vi "GOOP_DebugLogger.vi"(6 "ActivateDon'tCloseVI":bool, 7 "ActivateDebugging":bool, 8 "error in (no error)":errorcluster, 10 "Data":string, 11 "State":string) -> (0 "error out":errorcluster, 1 "Don'tCloseVI":bool, 3 "Debugging":bool)   [LabVIEW 2020]
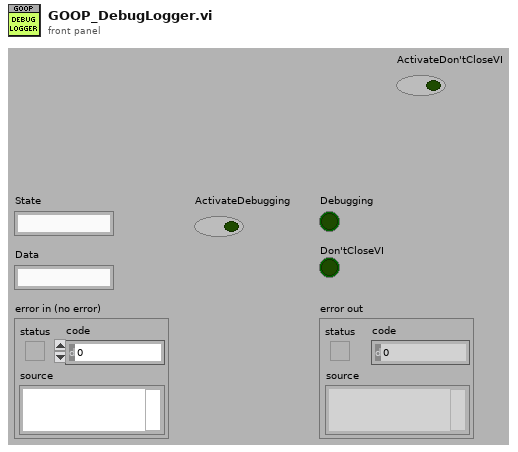
[diagram p1: front panel]
types:
  T1 = enum16{"open", "replace", "create", "open or create", "replace or create", "replace or create with confirmation"}
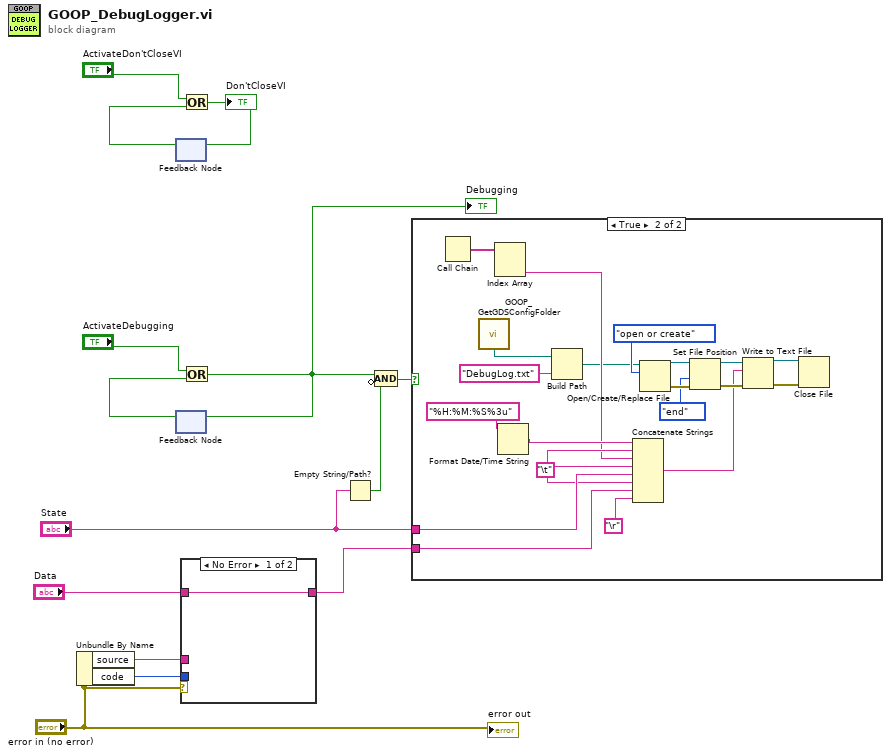
[diagram p0: block diagram]
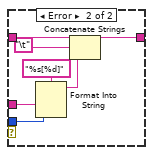
[diagram p2: hidden frame]
diagram:
  n1 = Unbundle By Name("error in (no error)") -> ("source"=w9:string, "code"=w8:i32)
  n2 = feedback #1() -> (w3:bool)  [unwired: 1 in]
  n3 = feedback #2() -> (w13:bool)  [unwired: 1 in]
  n4 = case shown="No Error" "error in (no error)" {
    tunnel: "Data" -> [w15 w22]
    tunnel: [w15 w20] -> w10
    tunnel: w9 -> [_ w19]
    tunnel: w8 -> [_ w18]
    frame No Error {
    }
    frame Error {
      n5 = Format Into String(format string="%s[%d]", w19, w18) -> (resulting string=w17:string)  [unwired: 2 in, 1 out]
      n6 = Concatenate Strings(w22, "\t", w17) -> (w20:string)
    }
  }
  n7 = Or(x="ActivateDon'tCloseVI", y=w3) -> (x .or. y?=w1:bool)
  "Don'tCloseVI" <- w1
  n8 = feedback-in #1(w1) -> ()
  n9 = Or(x="ActivateDebugging", y=w13) -> (x .or. y?=w6:bool)
  "Debugging" <- w6
  n10 = feedback-in #2(w6) -> ()
  n11 = Empty String/Path?(string/path="State") -> (empty?=w4:bool)
  n12 = Compound Arithmetic op=AND(w6, invert w4) -> (w5:bool)
  n13 = case shown="True" w5 {
    tunnel: "State" -> [_ w33]
    tunnel: w10 -> [_ w32]
    frame False {
    }
    frame True {
      w27 = "\t"
      n14 = Call Chain() -> (call chain=w29:string[])
      n15 = call "GOOP_GetGDSConfigFolder.vi"() -> ("GDSFolderPath"=w24:path)
      n16 = Index Array(array=w29) -> (element #2=w26:string)  [unwired: 2 in, 1 out]
      n17 = Format Date/Time String(time format string (%c)="%H:%M:%S%3u") -> (date/time string=w28:string)  [unwired: 2 in]
      n18 = Build Path(base path=w24, name or relative path="DebugLog.txt") -> (appended path=w23:path)
      n19 = Concatenate Strings(w28, w27, w26, w27, w33, w27, w32, "\r") -> (w30:string)
      n20 = Open/Create/Replace File(file path (use dialog)=w23, operation (0:open)=T1."open or create") -> (refnum out=w40:refnum<file>, error out=w41:errorcluster)  [unwired: 4 in, 1 out]
      n21 = Set File Position(refnum=w40, from (0:start)=enum16{"start", "end", "current"}."end", error in=w41) -> (refnum out=w37:refnum<file>, error out=w38:errorcluster)  [unwired: 1 in]
      n22 = Write to Text File(file (use dialog)=w37, text=w30, error in=w38) -> (refnum out=w35:refnum<file>, error out=w36:errorcluster)  [unwired: 1 in, 1 out]
      n23 = Close File(refnum=w35, error in=w36) -> ()  [unwired: 2 out]
    }
  }
  "error out" <- "error in (no error)"
